vi "Cosine연산.vi"() -> ()   [LabVIEW 2019]
panel:
  out "cos(x)":dbl
  in  "A":dbl
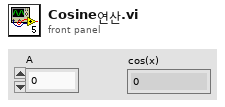
[diagram p1: front panel]
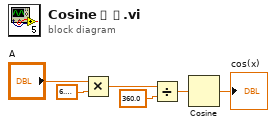
[diagram p0: block diagram]
diagram:
  n1 = Multiply(x="A", y=6.283185307179586) -> (x*y=w4:dbl)
  n2 = Divide(x=w4, y=360.0) -> (x/y=w1:dbl)
  n3 = Cosine(x=w1) -> (cos(x)=→"cos(x)":dbl)
